vi "Initialize.vi"(9 "Current Target":i32, 10 "Position":T1, 11 "Assassin in":refnum<class "Assassin.lvclass">) -> (3 "Assassin out":refnum<class "Assassin.lvclass">)   [LabVIEW 2015, in "Assassin.lvclass"]
uses:
  Assassin.lvclass
  Common/Position.ctl
  Assassin.lvclass/Assassin.ctl
  SubVIs/Read-Only Globals.vi
  SubVIs/Read-Only Stats.vi
  SubVIs/Globals (private).vi
  Square/Square.lvclass
  Common/Common.lvlib
panel:
  out "array w/ subset deleted":T1[](array[typedef])
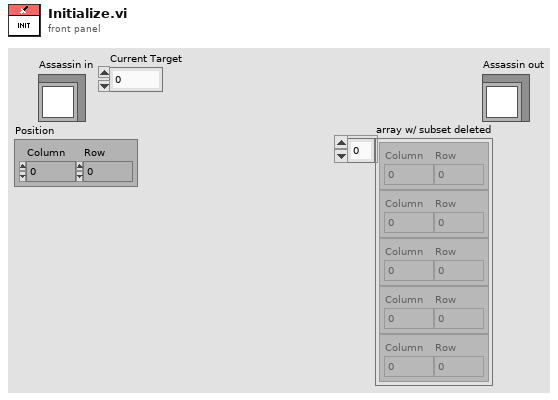
[diagram p1: front panel]
types:
  T1 = typedef "Common.lvlib/Position.ctl" = cluster{"Column":i32, "Row":i32}
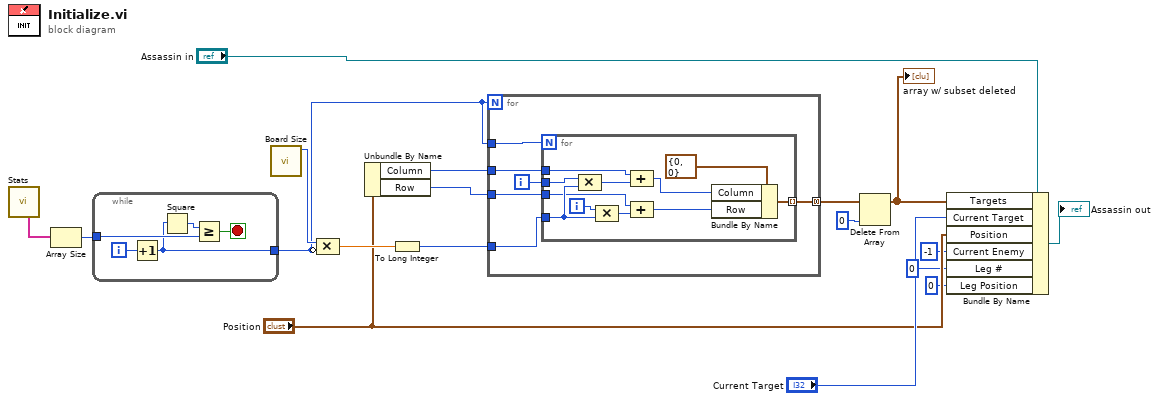
[diagram p0: block diagram]
diagram:
  n1 = call "Stats.vi"() -> ("Players"=w15:string[])  [unwired: 7 in, 4 out]
  n2 = Array Size(array=w15) -> (size(s)=w17:i32)
  n3 = while {
    tunnel: w17 -> [w21]
    tunnel: [w20] -> w13
    i -> [w23]
    stop <- w22 stop-if-true
    n4 = Increment(x=w23) -> (x+1=w20:i32)
    n5 = Square(x=w20) -> (x^2=w19:i32)
    n6 = Greater Or Equal?(x=w19, y=w21) -> (x >= y?=w22:bool)
  }
  n7 = call "Board Size.vi"() -> ("Board Size"=w16:i32)  [unwired: 11 in]
  n8 = Compound Arithmetic op=MULTIPLY(w16, invert w13) -> (w18:dbl)
  n9 = Unbundle By Name("Position") -> ("Column"=w11:i32, "Row"=w7:i32)
  n10 = To Long Integer(number=w18) -> (32bit integer=w8:i32)
  n11 = for {
    N: w13 -> [_]
    tunnel: w13 -> [w29]
    tunnel: w11 -> [w28]
    tunnel: [w26] -> w10 mode=concatenating
    tunnel: w8 -> [w25]
    tunnel: w7 -> [w24]
    i -> [w27]
    n12 = for {
      N: w29 -> [_]
      tunnel: w28 -> [w40]
      tunnel: w27 -> [w39]
      tunnel: [w30] -> w26 mode=indexing
      tunnel: w25 -> [w35]
      tunnel: w24 -> [w34]
      i -> [w36]
      n13 = Compound Arithmetic op=MULTIPLY(w39, w35) -> (w38:i32)
      n14 = Compound Arithmetic op=MULTIPLY(w36, w35) -> (w37:i32)
      n15 = Compound Arithmetic op=unknown(w40, w38) -> (w33:i32)
      n16 = Compound Arithmetic op=ADD(w34, w37) -> (w31:i32)
      n17 = Bundle By Name(cluster=T1 {"Column"=0, "Row"=0} ("Target"), "Column"=w33, "Row"=w31) -> (w30:T1)
    }
  }
  n18 = Delete From Array(array=w10, index=0) -> (array with subset deleted=w6:T1[])  [unwired: 1 in, 1 out]
  "array w/ subset deleted" <- w6
  n19 = Bundle By Name(cluster="Assassin in", "Targets"=w6, "Current Target"="Current Target", "Position"="Position", "Current Enemy"=-1, "Leg #"=0, "Leg Position"=0) -> (→"Assassin out":refnum<class "Assassin.lvclass">)
